vi "SetTile.vi"(8 "error in (no error)":errorcluster, 9 "Coordinates":T1, 10 "TileCode":u32) -> (0 "error out":errorcluster)   [LabVIEW 2019, in "RT_Game.lvlib" / "Engine.lvclass"]
doc: "Sets a Tile on the Screen.\nUse DrawTiles.vi to draw the tiles to the camera, once every Tile is set."
uses:
  Engine.lvclass
  Coordinate.ctl
  SetTileData.ctl
  MessageCluster.ctl
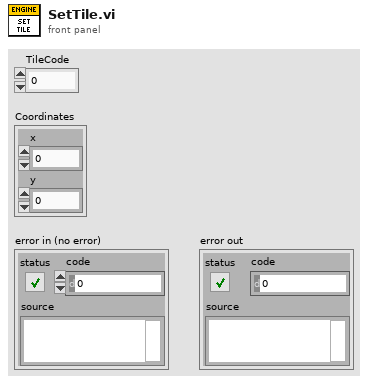
[diagram p1: front panel]
types:
  T1 = typedef "RT_Game.lvlib/Engine.lvclass/Coordinate.ctl" = cluster{"x":dbl, "y":dbl}
  T2 = typedef "RT_Game.lvlib/Engine.lvclass/MessageCluster.ctl" = cluster{"Message":string, "Data":variant}
  T3 = typedef "RT_Game.lvlib/Engine.lvclass/SetTileData.ctl" = cluster{"TileCode":u32, "Position":T1}
  T4 = typedef "RT_Game.lvlib/Engine.lvclass/Queues.ctl" = cluster{"MusicQueue":refnum<queue>, "TilesQueue":refnum<queue>, "SoundsQueue":refnum<queue>}
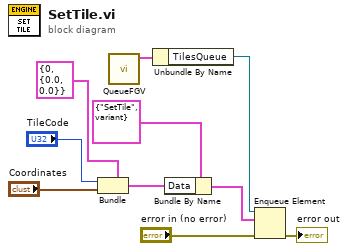
[diagram p0: block diagram]
diagram:
  n1 = Bundle(cluster=T3 {"TileCode"=0, "Position"={"x"=0.0, "y"=0.0}} ("SetTileData"), "TileCode"="TileCode", "Position"="Coordinates") -> (w10:T3)
  n2 = call "QueueFGV.vi"() -> ("Queues out"=w1:T4)  [unwired: 10 in, 1 out]
  n3 = Unbundle By Name(w1) -> ("TilesQueue"=w6:refnum<queue>)
  n4 = Bundle By Name(cluster=T2 {"Message"="SetTile", "Data"=variant} ("element"), "Data"=w10) -> (w8:T2)
  n5 = Enqueue Element(queue=w6, element=w8, error in (no error)="error in (no error)") -> (error out=→"error out":errorcluster)  [unwired: 1 in, 2 out]
